vi "Build Voltage XY Graph Data.vi"(6 "voltage below min":dbl format="%#_13g", 8 "maximum voltage":dbl, 9 "maximum speed":dbl, 10 "min voltage":dbl, 11 "min speed":dbl) -> (3 "XY data":cluster{dbl, dbl}[](array[cluster]))   [LabVIEW 2017, in "Engine Simulation Toolkit System Explorer.lvlib"]
uses:
  Engine Simulation Toolkit System Explorer.lvlib
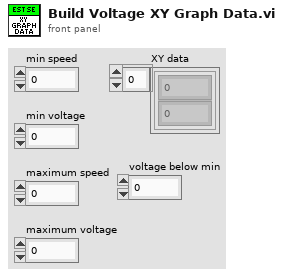
[diagram p1: front panel]
types:
  T1 = cluster{"min speed":dbl, "voltage below min":dbl}
  T2 = cluster{"maximum speed":dbl, "maximum voltage":dbl}
  T3 = cluster{"maximum speed":dbl, "maximum voltage":dbl}[]
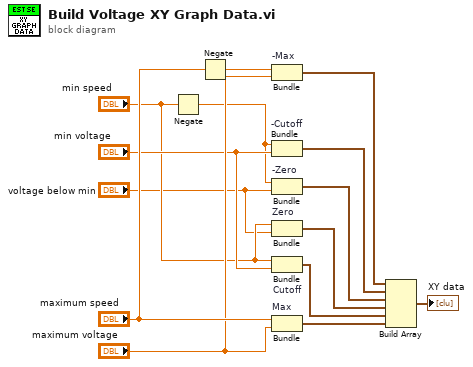
[diagram p0: block diagram]
diagram:
  n1 = Negate(x="min speed") -> (-x=w6:dbl)
  n2 = Negate(x="maximum speed") -> (-x=w10:dbl)
  n3 = Bundle "-Max"(w10, "maximum voltage"="maximum voltage") -> (w13:cluster{dbl, "maximum voltage":dbl})  [unwired: 1 in]
  n4 = Bundle "-Cutoff"(w6, "min voltage"="min voltage") -> (w7:cluster{dbl, "min voltage":dbl})  [unwired: 1 in]
  n5 = Bundle "-Zero"(w6, "voltage below min"="voltage below min") -> (w3:cluster{dbl, "voltage below min":dbl})  [unwired: 1 in]
  n6 = Bundle "Zero"("min speed"="min speed", "voltage below min"="voltage below min") -> (w2:T1)  [unwired: 1 in]
  n7 = Bundle "Cutoff"("min speed"="min speed", "min voltage"="min voltage") -> (w12:cluster{"min speed":dbl, "min voltage":dbl})  [unwired: 1 in]
  n8 = Bundle "Max"("maximum speed"="maximum speed", "maximum voltage"="maximum voltage") -> (w14:T2)  [unwired: 1 in]
  n9 = Build Array(w13, w7, w3, w2, w12, w14) -> (→"XY data":T3)
